vi "Helmholtz2D_Check Input_BC.vi"(8 "error in (no error)":errorcluster, 10 "Domain":T2={"x"={"start x"=0.0, "end x"=1.0, "# of x-points"=11}, "y"={"start y"=0.0, "end y"=1.0, "# of y-points"=11}}, 11 "Boundary Condition":cluster{"type":T1, "Value":dbl[]}[](array[cluster]) {"type" items=["Dirichlet", "Neumann"]}) -> (0 "error out":errorcluster)   [LabVIEW 2020, in "NI_PDE.lvlib"]
uses:
  <vilib>/gmath/NI_PDE.lvlib
  <vilib>/gmath/pde.llb/Common/PDE_BC Type.ctl
  <vilib>/gmath/pde.llb/Common/PDE_Error.ctl
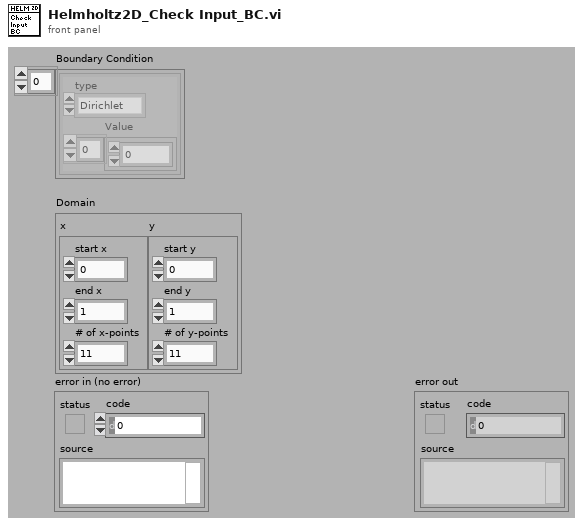
[diagram p1: front panel]
types:
  T1 = typedef "NI_PDE.lvlib/PDE_BC Type.ctl" = i32
  T2 = cluster{"x":cluster{"start x":dbl, "end x":dbl, "# of x-points":i32}, "y":cluster{"start y":dbl, "end y":dbl, "# of y-points":i32}}
  T3 = typedef "NI_PDE.lvlib/PDE_Error.ctl" = enum16{"No Error", "k is zero", "End point <= start point", "# of time steps < 2", "# of spatial points < 3", "# of grid < 1 for FEM", "# of boundary < 3 for FEM", "Incompatible RHS size", "Incompatible BC size", "Incompatible IC size", "PDE class conflict", "RHS class conflict", "Domain class conflict", "BC class conflict", "IC class conflict"}
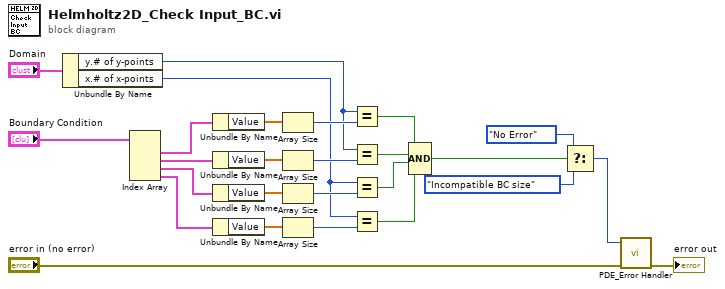
[diagram p0: block diagram]
diagram:
  n1 = Unbundle By Name("Domain") -> ("y.# of y-points"=w12:i32, "x.# of x-points"=w9:i32)
  n2 = Index Array(array="Boundary Condition") -> (element #1=w20:cluster{"type":T1, "Value":dbl[]}, element #2=w18:cluster{"type":T1, "Value":dbl[]}, element #3=w16:cluster{"type":T1, "Value":dbl[]}, element #4=w14:cluster{"type":T1, "Value":dbl[]})  [unwired: 4 in]
  n3 = Unbundle By Name(w20) -> ("Value"=w23:dbl[])
  n4 = Unbundle By Name(w18) -> ("Value"=w19:dbl[])
  n5 = Unbundle By Name(w16) -> ("Value"=w17:dbl[])
  n6 = Unbundle By Name(w14) -> ("Value"=w15:dbl[])
  n7 = Array Size(array=w23) -> (size(s)=w22:i32)
  n8 = Array Size(array=w19) -> (size(s)=w13:i32)
  n9 = Array Size(array=w17) -> (size(s)=w11:i32)
  n10 = Array Size(array=w15) -> (size(s)=w10:i32)
  n11 = Equal?(x=w12, y=w22) -> (x = y?=w8:bool)
  n12 = Equal?(x=w12, y=w13) -> (x = y?=w7:bool)
  n13 = Equal?(x=w9, y=w11) -> (x = y?=w6:bool)
  n14 = Equal?(x=w9, y=w10) -> (x = y?=w5:bool)
  n15 = Compound Arithmetic op=AND(w8, w7, w6, w5) -> (w4:bool)
  n16 = Select(t=PDE_Error."No Error" ("PDE error"), s=w4, f=PDE_Error."Incompatible BC size" ("PDE error")) -> (s? t:f=w3:T3)
  n17 = call <vilib>:"PDE_Error Handler.vi"("error in (no error)"="error in (no error)", "PDE error"=w3) -> ("error out"=→"error out":errorcluster)  [unwired: 9 out]
